vi "UserErrors.vi"(8 "error in (no error)":errorcluster, 11 "[error code] (0)":i32 format="%0.0f") -> (0 "error out":errorcluster)   [LabVIEW 2014]
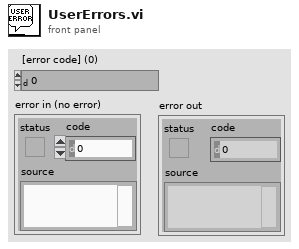
[diagram p1: front panel]
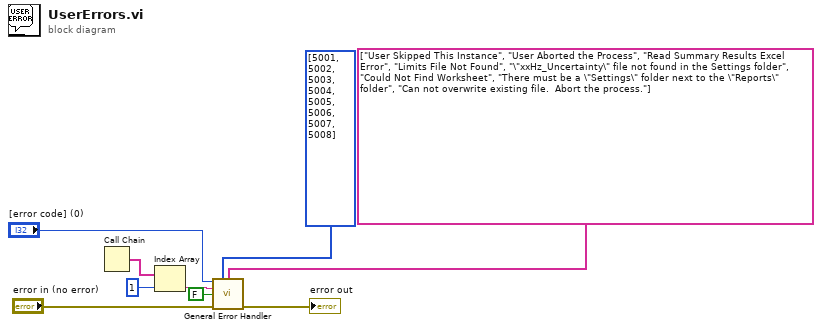
[diagram p0: block diagram]
diagram:
  n1 = Call Chain() -> (call chain=w4:string[])
  n2 = Index Array(array=w4, index=1) -> (element=w2:string)
  n3 = call <vilib>:"General Error Handler.vi"("[error code] (0)"="[error code] (0)", "[user-defined codes]"=i32[] [5001, 5002, 5003, 5004, 5005, 5006, 5007, 5008], "[user-defined descriptions]"=string[] ["User Skipped This Instance", "User Aborted the Process", "Read Summary Results Excel Error", "Limits File Not Found", "\"xxHz_Uncertainty\" file not found in the Settings folder", "Could Not Find Worksheet", "There must be a \"Settings\" folder next to the \"Reports\" folder", "Can not overwrite existing file.  Abort the process."], "[error source] (\" \")"=w2, "search ni.com link visible?(T)"=FALSE, "error in (no error)"="error in (no error)") -> ("error out"=→"error out":errorcluster)  [unwired: 5 in, 4 out]
